vi "ToyForStableDisplayOnGrabber.vi"() -> ()   [LabVIEW 2010]
panel:
  out "appended array":u32[](array[numeric])
  out "Array 3":u32[](array[numeric])
  in  "s":bool
  out "Array 2":u32[](array[numeric])
  in  "stop":bool
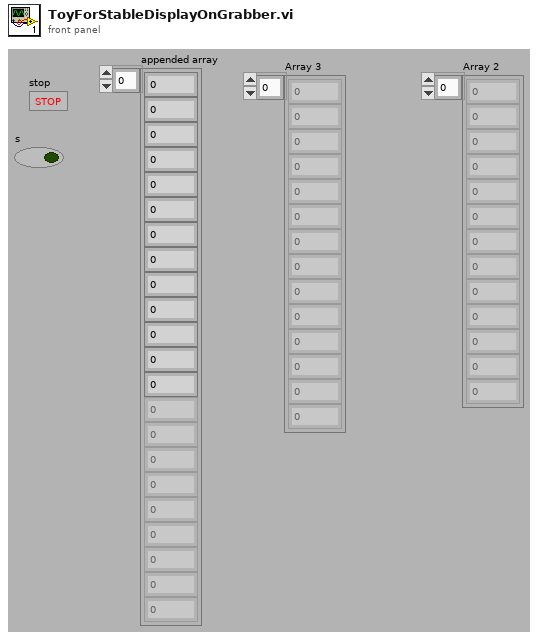
[diagram p1: front panel]
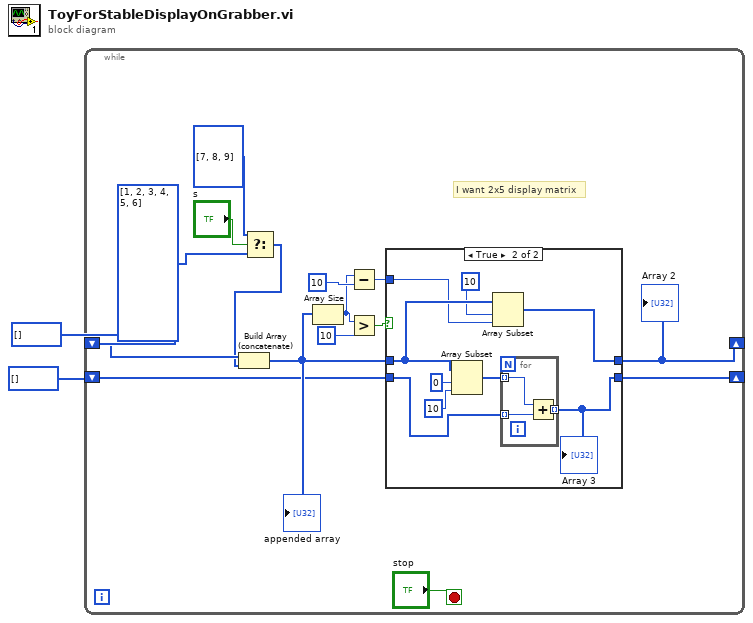
[diagram p0: block diagram]
diagram:
  n1 = while {
    shift-right: [w8] -> _
    shift-left: u32[] [] -> [w16]
    shift-right: [w4] -> _
    shift-left: u32[] [] -> [w3]
    stop <- "stop" stop-if-true
    # "I want 2x5 display matrix"
    n2 = Select(t=i32[] [7, 8, 9], s="s", f=i32[] [1, 2, 3, 4, 5, 6]) -> (s? t:f=w12:i32[])
    n3 = Build Array (concatenate)(w16, w12) -> (w11:u32[])
    "appended array" <- w11
    n4 = Array Size(array=w11) -> (size(s)=w6:i32)
    n5 = Subtract(x=w6, y=u8 10) -> (x-y=w5:i32)
    n6 = Greater?(x=w6, y=10) -> (0:w9:bool)
    n7 = case shown="True" w9 {
      tunnel: w11 -> [w19 w27]
      tunnel: [w19 w24] -> w8
      tunnel: w5 -> [_ w25]
      tunnel: [w18 w21] -> w4
      tunnel: w3 -> [w18 w20]
      frame False {
      }
      frame True {
        n8 = Array Subset(array=w27, index=0, length=10) -> (w22:u32[])
        n9 = Array Subset(array=w27, index=10, length=w25) -> (w24:u32[])
        n10 = for {
          tunnel: w22 -> [w31] mode=indexing
          tunnel: [w30] -> w21 mode=indexing
          tunnel: w20 -> [w29] mode=indexing
          n11 = Add(x=w31, y=w29) -> (x+y=w30:u32)
        }
        "Array 3" <- w21
      }
    }
    "Array 2" <- w8
  }
